vi "Send Impedance Analyzer Command.vi"(8 "error in (no error)":errorcluster, 10 "write buffer":string, 11 "VISA resource name":refnum<visa-resource-name>) -> (0 "error out":errorcluster, 3 "VISA resource name out":refnum<visa-resource-name>)   [LabVIEW 2017]
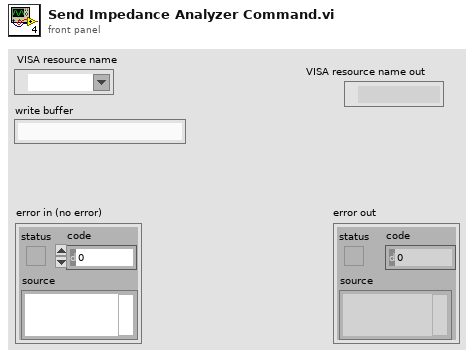
[diagram p1: front panel]
types:
  T1 = typedef "Semaphore RefNum" = refnum<k1>
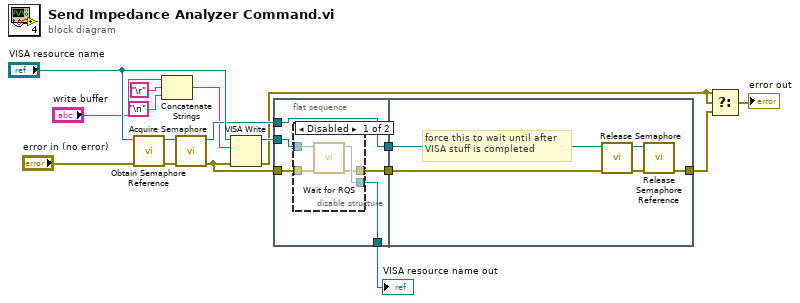
[diagram p0: block diagram]
diagram:
  n1 = call <vilib>:"Obtain Semaphore Reference.vi"("error in (no error)"="error in (no error)", "name (unnamed)"="VISA resource name") -> ("error out"=w16:errorcluster, "semaphore"=w17:T1)  [unwired: 1 in, 3 out]
  n2 = Concatenate Strings("write buffer", "\r", "\n") -> (w3:string)
  n3 = call <vilib>:"Acquire Semaphore.vi"("error in (no error)"=w16, "semaphore"=w17) -> ("error out"=w12:errorcluster, "semaphore out"=w14:T1)  [unwired: 1 in, 3 out]
  n4 = VISA Write(VISA resource name="VISA resource name", write buffer=w3, error in (no error)=w12) -> (VISA resource name out=w2:refnum<visa-resource-name>, error out=w1:errorcluster)  [unwired: 1 out]
  n5 = flat-sequence {
    tunnel: w12 -> [w19]
    tunnel: w14 -> [w22]
    tunnel: [w22] -> w9
    tunnel: [w18] -> w8
    tunnel: w2 -> [w21]
    tunnel: [w20] -> w7
    tunnel: [w30] -> w11
    tunnel: w9 -> [w33]
    tunnel: w8 -> [w29]
    frame #0 {
      n6 = disable-structure shown="Disabled" {
        disable-tunnel: w21 -> [w26 w28]
        disable-tunnel: [w25 w28] -> w20
        disable-tunnel: w19 -> [w24 w27]
        disable-tunnel: [w23 w27] -> w18
        frame Disabled {
          n7 = call <vilib>:"Wait for RQS.vi"("error in (no error)"=w24, "VISA resource name"=w26) -> ("error out"=w23:errorcluster, "VISA resource name out"=w25:refnum<visa-resource-name>)  [unwired: 7 in, 1 out]
        }
        frame Enabled {
        }
      }
    }
    frame #1 {
      # "force this to wait until after \nVISA stuff is completed"
      n8 = call <vilib>:"Release Semaphore.vi"("error in (no error)"=w29, "semaphore"=w33) -> ("error out"=w31:errorcluster, "semaphore out"=w32:T1)  [unwired: 4 out]
      n9 = call <vilib>:"Release Semaphore Reference.vi"("error in (no error)"=w31, "semaphore"=w32) -> ("error out"=w30:errorcluster)  [unwired: 9 out]
    }
  }
  n10 = Select(t=w1, s=w1, f=w11) -> (s? t:f=→"error out":errorcluster)
  "VISA resource name out" <- w7
